vi "CallbackSystemExec.vi"(8 "error in (no error)":errorcluster, 9 "Caller Events":T1, 10 "Working directory":path, 11 "Command":string) -> (0 "error out":errorcluster, 2 "Standard Error":string, 3 "Standard Out":string)   [LabVIEW 2018, in "callback-system-exec.lvlib"]
uses:
  callback-system-exec.lvlib
  3b7a8aed-5023-428e-8bf6-ff0110012a15.vi
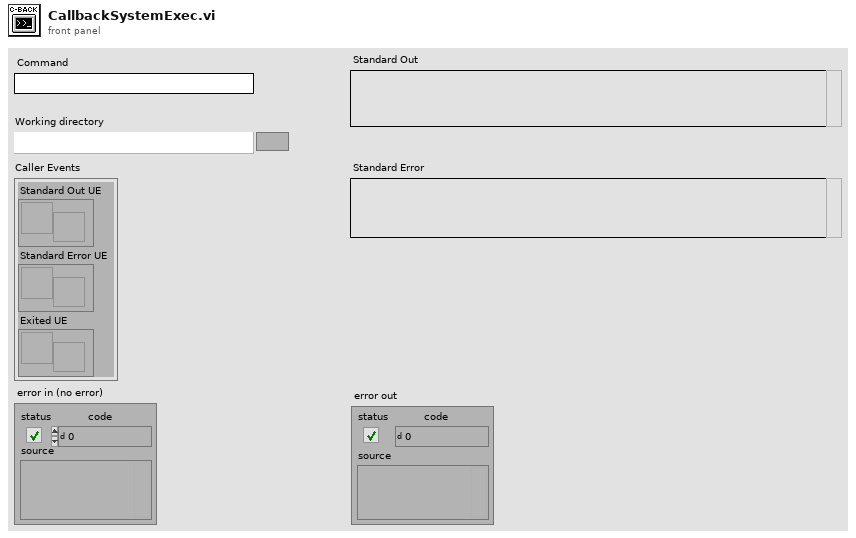
[diagram p1: front panel]
types:
  T1 = cluster{"Standard Out UE":refnum<user-event>, "Standard Error UE":refnum<user-event>, "Exited UE":refnum<user-event>}
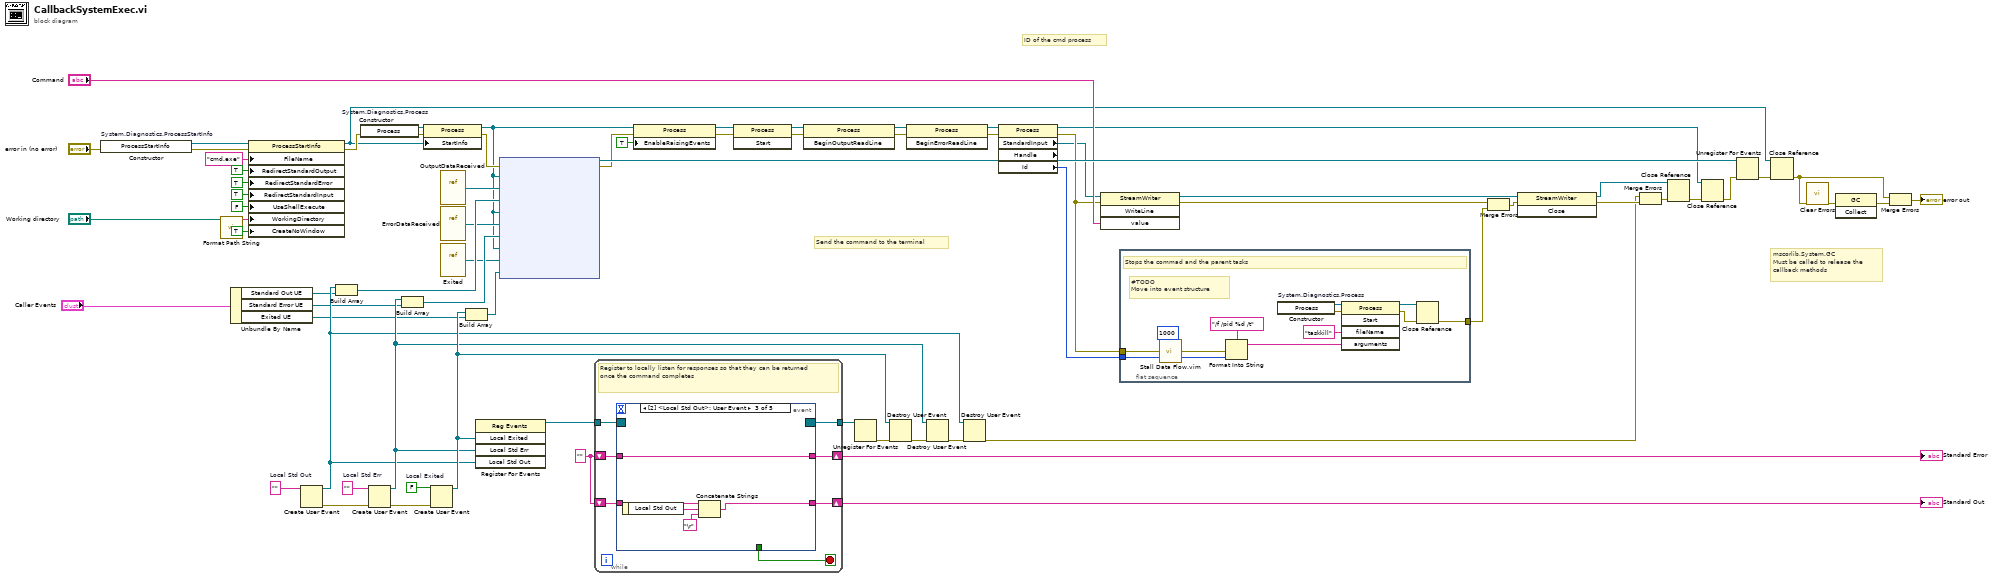
[diagram p0: block diagram]
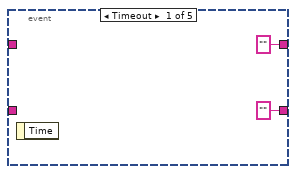
[diagram p2: hidden frame]
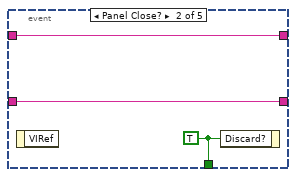
[diagram p3: hidden frame]
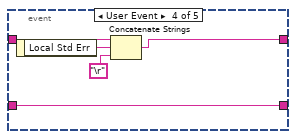
[diagram p4: hidden frame]
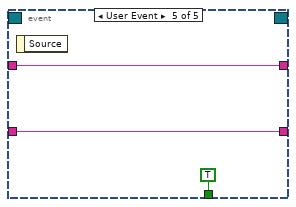
[diagram p5: hidden frame]
diagram:
  w19 = ""
  w35 = FALSE  # Local Exited
  w36 = ""  # Local Std Err
  w37 = ""  # Local Std Out
  # "ID of the cmd process"
  # "mscorlib.System.GC\nMust be called to release the \ncallback methods"
  # "Send the command to the terminal"
  n1 = constructor on="System.Diagnostics.ProcessStartInfo" class="ProcessStartInfo"(error in="error in (no error)") -> (reference out=w73:refnum<k24>, error out=w72:errorcluster)  [unwired: 2 in, 1 out]
  n2 = call "Format Path String.vi"("Path in"="Working directory") -> ("String out"=w65:string)  [unwired: 10 in]
  n3 = Unbundle By Name("Caller Events") -> ("Standard Out UE"=w17:refnum<user-event>, "Standard Error UE"=w16:refnum<user-event>, "Exited UE"=w15:refnum<user-event>)
  n4 = property class="ProcessStartInfo"(reference=w73, error in=w72, "FileName"="cmd.exe", "RedirectStandardOutput"=TRUE, "RedirectStandardError"=TRUE, "RedirectStandardInput"=TRUE, "UseShellExecute"=FALSE, "WorkingDirectory"=w65, "CreateNoWindow"=TRUE) -> (reference out=w2:refnum<k24>, error out=w61:errorcluster)
  n5 = Create User Event(user event datatype=w37) -> (user event=w24:refnum<user-event>, error out=w14:errorcluster)  [unwired: 1 in]
  n6 = Build Array(w24, w17) -> (w33:refnum<user-event>[])
  n7 = constructor on="System.Diagnostics.Process" class="Process"(error in=w61) -> (reference out=w62:refnum<k24>, error out=w63:errorcluster)  [unwired: 2 in, 1 out]
  n8 = Create User Event(user event datatype=w36, error in=w14) -> (user event=w25:refnum<user-event>, error out=w13:errorcluster)
  n9 = Build Array(w25, w16) -> (w34:refnum<user-event>[])
  n10 = property class="Process"(reference=w62, error in=w63, "StartInfo"=w2) -> (reference out=w20:refnum<k24>, error out=w60:errorcluster)
  n11 = Create User Event(user event datatype=w35, error in=w13) -> (user event=w26:refnum<user-event>)  [unwired: 1 out]
  n12 = vi-ref "OutputDataReceived.vi"() -> ("vi reference"=w23:refnum<vi>)
  n13 = vi-ref "ErrorDataReceived.vi"() -> ("vi reference"=w22:refnum<vi>)
  n14 = vi-ref "Exited.vi"() -> ("vi reference"=w21:refnum<vi>)
  n15 = Build Array(w26, w15) -> (w5:refnum<user-event>[])
  n16 = register-events(w26, w25, w24) -> (reference out=w32:refnum<event-registration>)  [unwired: 2 in, 1 out]
  n17 = node(w60, w20, w23, w33, w20, w22, w34, w20, w21, w5) -> (w43:refnum<k27>, w41:errorcluster)  [unwired: 1 in]
  n18 = while {
    tunnel: w32 -> [w80]
    tunnel: [w79] -> w31
    shift-right: [w77] -> w12
    shift-left: w19 -> [w78]
    shift-right: [w76] -> w11
    shift-left: w19 -> [w75]
    stop <- w81 stop-if-true
    # "Register to locally listen for responses so that they can be returned once the command completes"
    n19 = event shown="[2] <Local Std Out>: User Event" {
      selector: w80 -> [_ _ _ _ _]
      dyn-events: [_ _ _ _ _] -> w79
      timeout: _ -> [_ _ _ _ _]
      tunnel: [_ w86 _ _ TRUE] -> w81
      tunnel: w78 -> [_ w85 w90 w96 w99]
      tunnel: ["" w85 w88 w96 w99] -> w77
      tunnel: ["" w84 w87 w92 w97] -> w76
      tunnel: w75 -> [_ w84 w87 w94 w97]
      event Timeout {
        n20 = event-data() -> ()  [unwired: 1 in, 1 out]
      }
      event Panel Close? {
        w86 = TRUE
        n21 = event-data() -> ()  [unwired: 1 in, 1 out]
        n22 = event-data("Discard?"=w86) -> ()  [unwired: 1 in, 1 out]
      }
      event User Event {
        n23 = event-data() -> ("Local Std Out"=w89:string)  [unwired: 1 in]
        n24 = Concatenate Strings(w90, w89, "\r") -> (w88:string)
      }
      event User Event {
        n25 = event-data() -> ("Local Std Err"=w93:string)  [unwired: 1 in]
        n26 = Concatenate Strings(w94, w93, "\r") -> (w92:string)
      }
      event User Event {
        n27 = event-data() -> ()  [unwired: 1 in, 1 out]
      }
    }
  }
  "Standard Out" <- w12
  "Standard Error" <- w11
  n28 = property class="Process"(reference=w20, error in=w41, "EnableRaisingEvents"=TRUE) -> (reference out=w57:refnum<k24>, error out=w58:errorcluster)
  n29 = invoke class="Process" method="Start"(reference=w57, error in=w58) -> (reference out=w55:refnum<k24>, error out=w56:errorcluster)  [unwired: 1 in, 1 out]
  n30 = invoke class="Process" method="BeginOutputReadLine"(reference=w55, error in=w56) -> (reference out=w53:refnum<k24>, error out=w54:errorcluster)  [unwired: 1 in, 1 out]
  n31 = Unregister For Events(event registration refnum=w31) -> (error out=w30:errorcluster)  [unwired: 1 in]
  n32 = Destroy User Event(user event=w26, error in=w30) -> (error out=w28:errorcluster)
  n33 = invoke class="Process" method="BeginErrorReadLine"(reference=w53, error in=w54) -> (reference out=w52:refnum<k24>, error out=w51:errorcluster)  [unwired: 1 in, 1 out]
  n34 = Destroy User Event(user event=w25, error in=w28) -> (error out=w27:errorcluster)
  n35 = Destroy User Event(user event=w24, error in=w27) -> (error out=w29:errorcluster)
  n36 = property class="Process" props=["StandardInput", "Handle", "Id"](reference=w52, error in=w51) -> (reference out=w4:refnum<k24>, error out=w8:errorcluster, "StandardInput"=w7:refnum<k24>, "Id"=w1:i32)  [unwired: 1 out]
  n37 = invoke class="StreamWriter" method="WriteLine"(reference=w7, error in=w8, "value"="Command") -> (reference out=w6:refnum<k24>, error out=w9:errorcluster)  [unwired: 1 in, 2 out]
  n38 = flat-sequence {
    tunnel: w8 -> [w111]
    tunnel: [w110] -> w3
    tunnel: w1 -> [w109]
    frame #0 {
      # "#TODO\nMove into event structure"
      # "Stops the commad and the parent tasks"
      n39 = call "Stall Data Flow.vim"("value in"=w111, "milliseconds to wait"=u32 1000) -> ("value out"=w103:errorcluster)  [unwired: 1 out]
      n40 = Format Into String(format string="/f /pid %d /t", error in=w103, w109) -> (resulting string=w100:string)  [unwired: 1 in, 1 out]
      n41 = constructor on="System.Diagnostics.Process" class="Process"() -> (reference out=w106:refnum<k24>, error out=w107:errorcluster)  [unwired: 3 in, 1 out]
      n42 = invoke class="Process" method="Start"(reference=w106, error in=w107, "fileName"="taskkill", "arguments"=w100) -> (reference out=w104:refnum<k24>, error out=w105:errorcluster)  [unwired: 1 in, 3 out]
      n43 = Close Reference(reference=w104, error in (no error)=w105) -> (error out=w110:errorcluster)
    }
  }
  n44 = Merge Errors(w9, w3) -> (w10:errorcluster)
  n45 = invoke class="StreamWriter" method="Close"(reference=w6, error in=w10) -> (reference out=w49:refnum<k24>, error out=w50:errorcluster)  [unwired: 1 in, 1 out]
  n46 = Merge Errors(w29, w50) -> (w45:errorcluster)
  n47 = Close Reference(reference=w49, error in (no error)=w45) -> (error out=w48:errorcluster)
  n48 = Close Reference(reference=w4, error in (no error)=w48) -> (error out=w47:errorcluster)
  n49 = Unregister For Events(event registration refnum=w43, error in=w47) -> (error out=w46:errorcluster)
  n50 = Close Reference(reference=w2, error in (no error)=w46) -> (error out=w38:errorcluster)
  n51 = call <vilib>:"Clear Errors.vi"("error in (no error)"=w38) -> ("error out"=w44:errorcluster)  [unwired: 5 in, 1 out]
  n52 = invoke class="GC" method="Collect"(error in=w44) -> (error out=w40:errorcluster)  [unwired: 2 in, 2 out]
  n53 = Merge Errors(w38, w40) -> (→"error out":errorcluster)
